vi "RemoteControl.Remote Client.vi"(5 "Port":u16=6341, 6 "timeout (ms) [500]":i32=500, 7 "address":string, 8 "error in (no error)":errorcluster, 9 "Data":variant, 10 "Command":string, 11 "RemoteControl in":refnum<class "RemoteControl.lvclass">) -> (0 "error out":errorcluster, 1 "Data out":variant, 2 "Command out":string, 3 "RemoteControl out":refnum<class "RemoteControl.lvclass">)   [LabVIEW 2019, in "RemoteControl.lvclass"]
uses:
  RemoteControl.lvclass
panel:
  # "Simple Client"
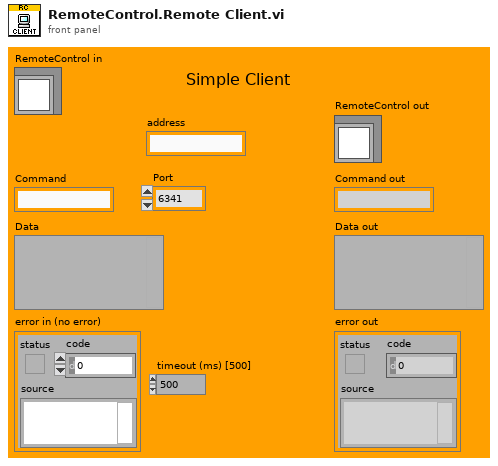
[diagram p1: front panel]
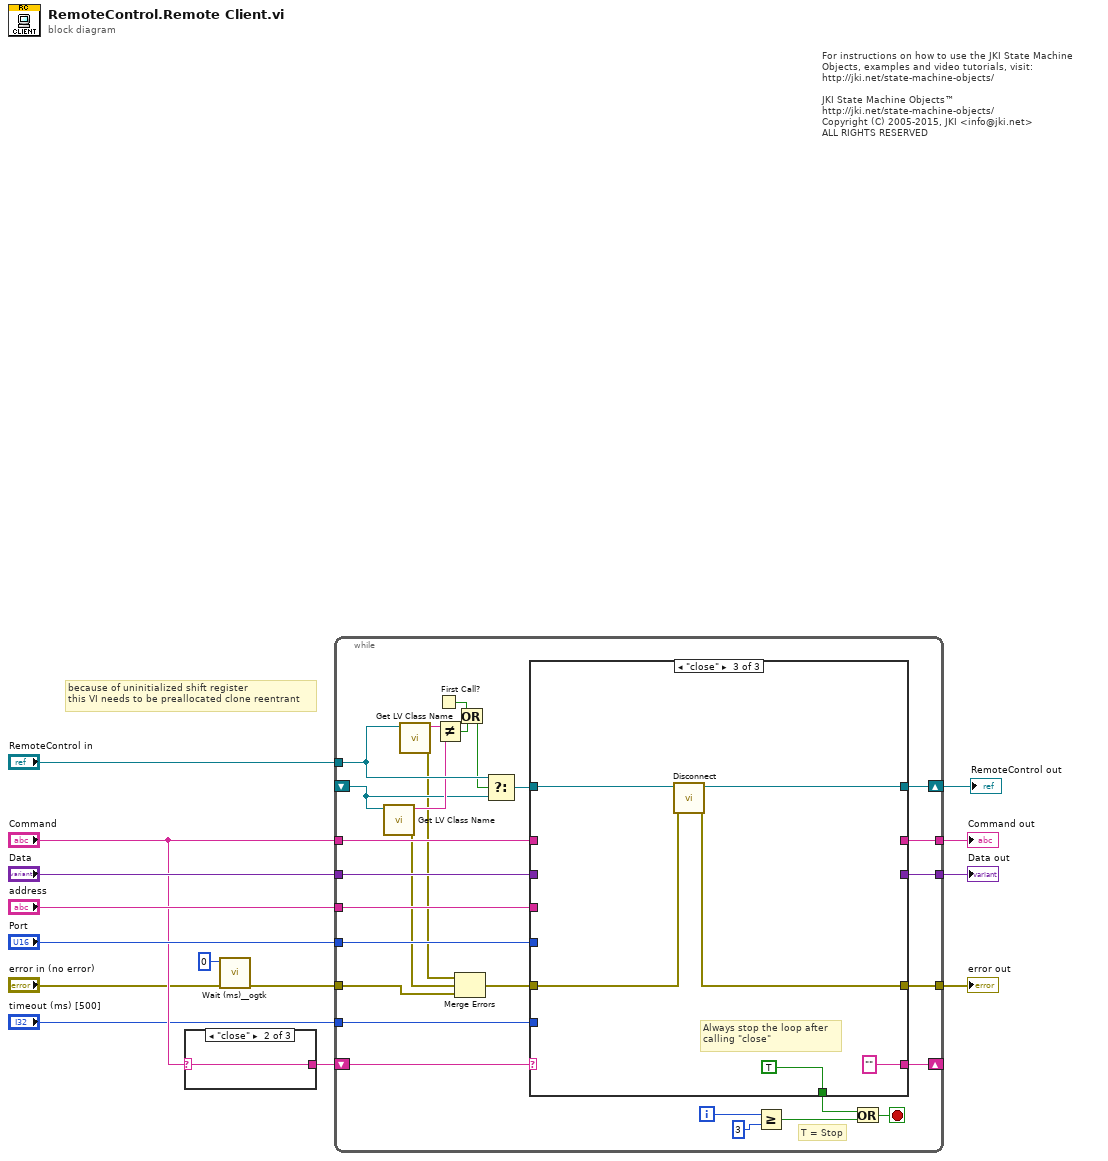
[diagram p0: block diagram]
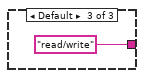
[diagram p3: hidden frame]
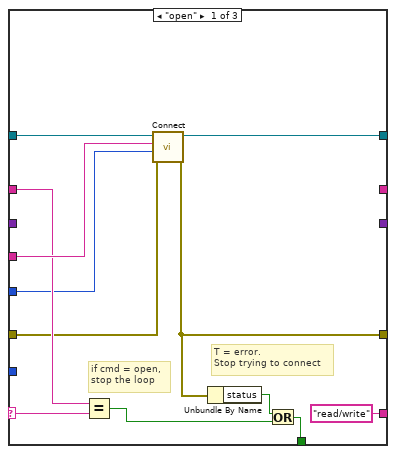
[diagram p4: hidden frame]
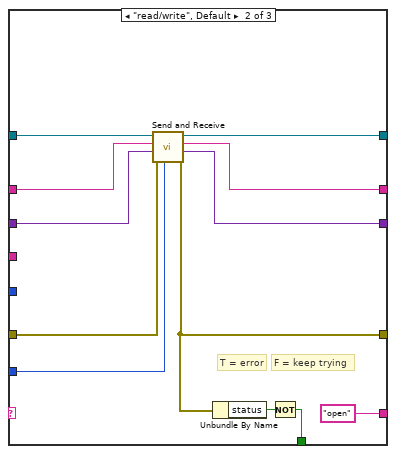
[diagram p5: hidden frame]
diagram:
  # "because of uninitialized shift register\nthis VI needs to be preallocated clone reentrant"
  # "For instructions on how to use the JKI State Machine Objects, examples and video tutorials, visit:\nhttp://jki.net/state-machine-objects/\n\nJKI State Machine Objects™\nhttp://jki.net/state-machine-objects/\nCopyright (C) 2005-2015, JKI <info@jki.net>\nALL RIGHTS RESERVED"
  n1 = case shown="\"close\"" "Command" {
    selector: "Command" -> [w15 w16 _]
    tunnel: [w15 w16 "read/write"] -> w6
    frame "open" {
    }
    frame "close" {
    }
    frame Default {
    }
  }
  n2 = call <userlib>:"Wait (ms)__ogtk.vi"("error in (no error)"="error in (no error)", "milliseconds to wait"=u32 0) -> ("error out"=w5:errorcluster)  [unwired: 8 in, 1 out]
  n3 = while {
    tunnel: "Port" -> [w43]
    tunnel: "address" -> [w42]
    shift-right: [w45] -> w13
    shift-left: _ -> [w20]
    shift-right: [w38] -> _
    shift-left: w6 -> [w31]
    tunnel: "RemoteControl in" -> [w30]
    tunnel: "Data" -> [w41]
    tunnel: [w39] -> w8
    tunnel: "Command" -> [w32]
    tunnel: [w40] -> w9
    tunnel: w5 -> [w22]
    tunnel: [w44] -> w14
    tunnel: "timeout (ms) [500]" -> [w18]
    i -> [w37]
    stop <- w33 stop-if-true
    # "T = Stop"
    n4 = call <vilib>:"Get LV Class Name.vi"("object"=w20) -> ("error out"=w23:errorcluster, "class name"=w24:string)  [unwired: 9 in]
    n5 = call <vilib>:"Get LV Class Name.vi"("object"=w30) -> ("error out"=w19:errorcluster, "class name"=w29:string)  [unwired: 9 in]
    n6 = First Call?() -> (First Call?: T/F=w28:bool)
    n7 = Not Equal?(x=w29, y=w24) -> (x != y?=w27:bool)
    n8 = Merge Errors(w19, w23, w22) -> (w21:errorcluster)
    n9 = Or(x=w28, y=w27) -> (x .or. y?=w25:bool)
    n10 = Select(t=w30, s=w25, f=w20) -> (s? t:f=w26:refnum<class "RemoteControl.lvclass">)
    n11 = case shown="\"close\"" w31 {
      selector: w31 -> [w54 _ _]
      tunnel: [w56 w69 w75] -> w45
      tunnel: [w46 w63 w70] -> w44
      tunnel: w43 -> [w48 _ _]
      tunnel: w21 -> [w49 w64 w71]
      tunnel: w42 -> [w57 _ _]
      tunnel: w41 -> [_ w58 _]
      tunnel: w32 -> [w53 w61 _]
      tunnel: [_ w62 _] -> w40
      tunnel: [_ w68 _] -> w39
      tunnel: ["read/write" "open" ""] -> w38
      tunnel: [w51 w65 TRUE] -> w35
      tunnel: w26 -> [w47 w60 w72]
      tunnel: w18 -> [_ w59 _]
      frame "open" {
        # "if cmd = open,\nstop the loop"
        # "T = error.\nStop trying to connect"
        n12 = Equal?(x=w53, y=w54) -> (x = y?=w52:bool)
        n13 = call "Connect.vi"("error in (no error)"=w49, "Port"=w48, "address"=w57, "RemoteControl in"=w47) -> ("error out"=w46:errorcluster, "RemoteControl out"=w56:refnum<class "RemoteControl.lvclass">)  [unwired: 6 in]
        n14 = Unbundle By Name(w46) -> ("status"=w50:bool)
        n15 = Or(x=w50, y=w52) -> (x .or. y?=w51:bool)
      }
      frame "read/write", Default {
        # "F = keep trying"
        # "T = error"
        n16 = call "Send and Receive.vi"("timeout (ms) [500]"=w59, "error in (no error)"=w64, "Data"=w58, "Command"=w61, "RemoteControl in"=w60) -> ("error out"=w63:errorcluster, "Data out"=w68:variant, "Command out"=w62:string, "RemoteControl out"=w69:refnum<class "RemoteControl.lvclass">)  [unwired: 3 in]
        n17 = Unbundle By Name(w63) -> ("status"=w66:bool)
        n18 = Not(x=w66) -> (.not. x?=w65:bool)
      }
      frame "close" {
        # "Always stop the loop after\ncalling \"close\""
        n19 = call "Disconnect.vi"("error in (no error)"=w71, "RemoteControl in"=w72) -> ("error out"=w70:errorcluster, "RemoteControl out"=w75:refnum<class "RemoteControl.lvclass">)  [unwired: 8 in]
      }
    }
    n20 = Greater Or Equal?(x=w37, y=3) -> (x >= y?=w34:bool)
    n21 = Or(x=w35, y=w34) -> (x .or. y?=w33:bool)
  }
  "RemoteControl out" <- w13
  "error out" <- w14
  "Data out" <- w8
  "Command out" <- w9
